vi "Set XScale Format.vi"(5 "timestamp eq 0":bool, 9 "Waveform Graph":refnum<vi>) -> ()   [LabVIEW 2020, in "TdmsFileViewer.lvlib"]
uses:
  TdmsFileViewer.lvlib
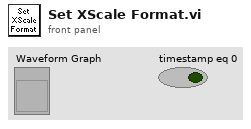
[diagram p1: front panel]
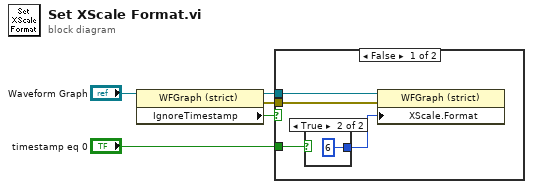
[diagram p0: block diagram]
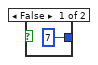
[diagram p2: hidden frame]
diagram:
  n1 = property class="WFGraph (strict)"(reference="Waveform Graph") -> (reference out=w1:refnum<vi>, error out=w5:errorcluster, "IgnoreTimestamp"=w3:bool)  [unwired: 1 in]
  n2 = case shown="False" w3 {
    tunnel: "timestamp eq 0" -> [w7 _]
    tunnel: w1 -> [w6 _]
    tunnel: w5 -> [w9 _]
    frame False {
      n3 = case shown="True" w7 {
        tunnel: [u8 7 u8 6] -> w8
        frame False {
        }
        frame True {
        }
      }
      n4 = property on="Property Node" class="WFGraph (strict)"(reference=w6, error in=w9, "XScale.Format"=w8) -> ()  [unwired: 2 out]
    }
    frame True {
    }
  }
